vi "integrand_of_2.15_m.vi"(1 "Initialise":bool, 2 "z*":dbl format="%.4f", 3 "y*":dbl format="%.2f", 4 "x*":dbl format="%.2f") -> (0 "Integrand":dbl format="%.2f")   [LabVIEW 2010]
uses:
  xw_correction_global_m.vi
panel:
  out "Ji":dbl[](array[numeric]) format="%.2f"
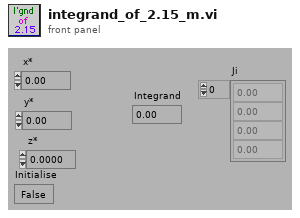
[diagram p1: front panel]
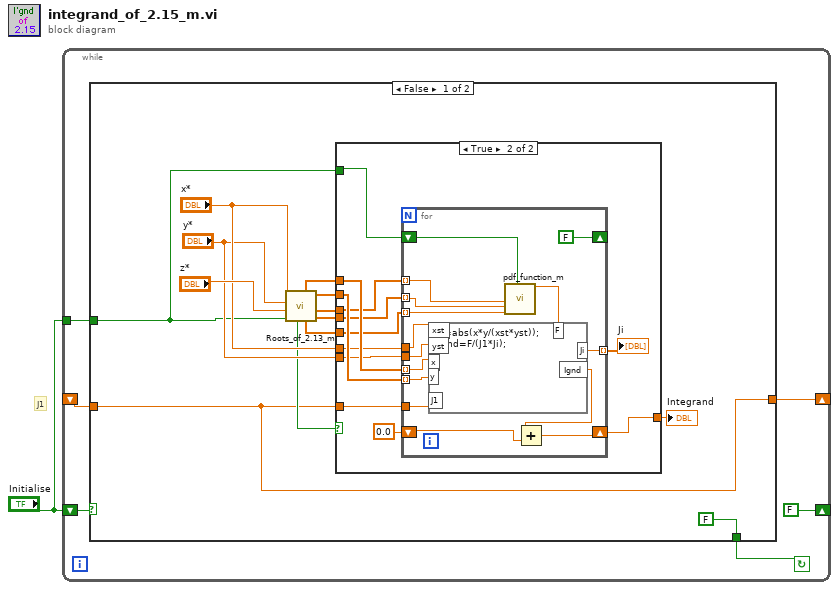
[diagram p0: block diagram]
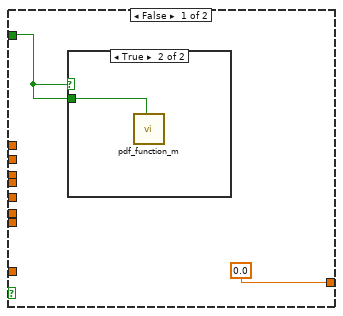
[diagram p2: hidden frame]
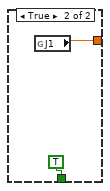
[diagram p4: hidden frame]
diagram:
  # "J1"
  n1 = while {
    shift-left: _ -> [w3]
    shift-right: [w2] -> _
    tunnel: "Initialise" -> [w4]
    shift-left: "Initialise" -> [w5]
    shift-right: [FALSE] -> _
    stop <- w7 continue-if-true
    n2 = case shown="False" w5 {
      tunnel: [FALSE TRUE] -> w7
      tunnel: w4 -> [w9 _]
      tunnel: w3 -> [w8 _]
      tunnel: [w8 w52] -> w2
      frame False {
        n3 = call "Roots_of_2.13_m.vi"("Initialise"=w9, "z"="z*", "y*"="y*", "x*"="x*") -> ("v"=w14:dbl[], "u"=w15:dbl[], "y"=w18:dbl[], "w"=w13:dbl[], "x"=w19:dbl[], "Roots exist"=w12:bool)  [unwired: 2 out]
        n4 = case shown="True" w12 {
          tunnel: w19 -> [_ w34]
          tunnel: w18 -> [_ w33]
          tunnel: "x*" -> [_ w32]
          tunnel: "y*" -> [_ w31]
          tunnel: w15 -> [_ w30]
          tunnel: w14 -> [_ w29]
          tunnel: w13 -> [_ w28]
          tunnel: [0.0 w27] -> w11
          tunnel: w8 -> [_ w25]
          tunnel: w9 -> [w21 w24]
          frame False {
            n5 = case shown="True" w21 {
              tunnel: w21 -> [_ w23]
              frame False {
              }
              frame True {
                n6 = call "pdf_function_m.vi"("Initialise"=w23) -> ()  [unwired: 8 in, 11 out]
              }
            }
          }
          frame True {
            n7 = for {
              tunnel: w30 -> [w50] mode=indexing
              tunnel: w29 -> [w49] mode=indexing
              tunnel: w28 -> [w48] mode=indexing
              tunnel: w32 -> [w46]
              tunnel: w31 -> [w45]
              tunnel: w33 -> [w43] mode=indexing
              tunnel: w34 -> [w44] mode=indexing
              shift-right: [w40] -> w27
              shift-left: 0.0 -> [w42]
              tunnel: [w39] -> w26 mode=indexing
              tunnel: w25 -> [w38]
              shift-right: [FALSE ("Initialise")] -> _
              shift-left: w24 -> [w37]
              n8 = call "pdf_function_m.vi"("u"=w50, "v"=w49, "w"=w48, "Initialise"=w37) -> ("F"=w47:dbl)  [unwired: 5 in, 10 out]
              n9 = formula code="Ji=abs(x*y/(xst*yst));\nIgnd=F/(J1*Ji);"("F"=w47, "xst"=w46, "yst"=w45, "x"=w44, "y"=w43, "J1"=w38) -> ("Ji"=w39:dbl, "Ignd"=w41:dbl)
              n10 = Add(x=w41, y=w42) -> (x+y=w40:dbl)
            }
            "Ji" <- w26
          }
        }
        "Integrand" <- w11
      }
      frame True {
        n11 = global read "xw_correction_global_m.vi" "J1"() -> (w52:dbl)
      }
    }
  }
